vi "测试类型1自动测试一组.vi"() -> ()   [LabVIEW 2010]
uses:
  全局量/试验配置信息.vi
  全局量/自动测试结果.vi
panel:
  out "EVENT_KEY":string
  out "bRece":bool
  out "bSend":bool
  out "第几个":i32
  in  "测试值":dbl
  out "bStop":bool
  out "数据组数":i32
  out "第几组":i32
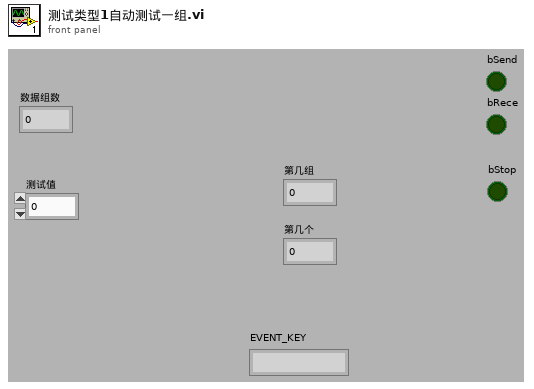
[diagram p1: front panel]
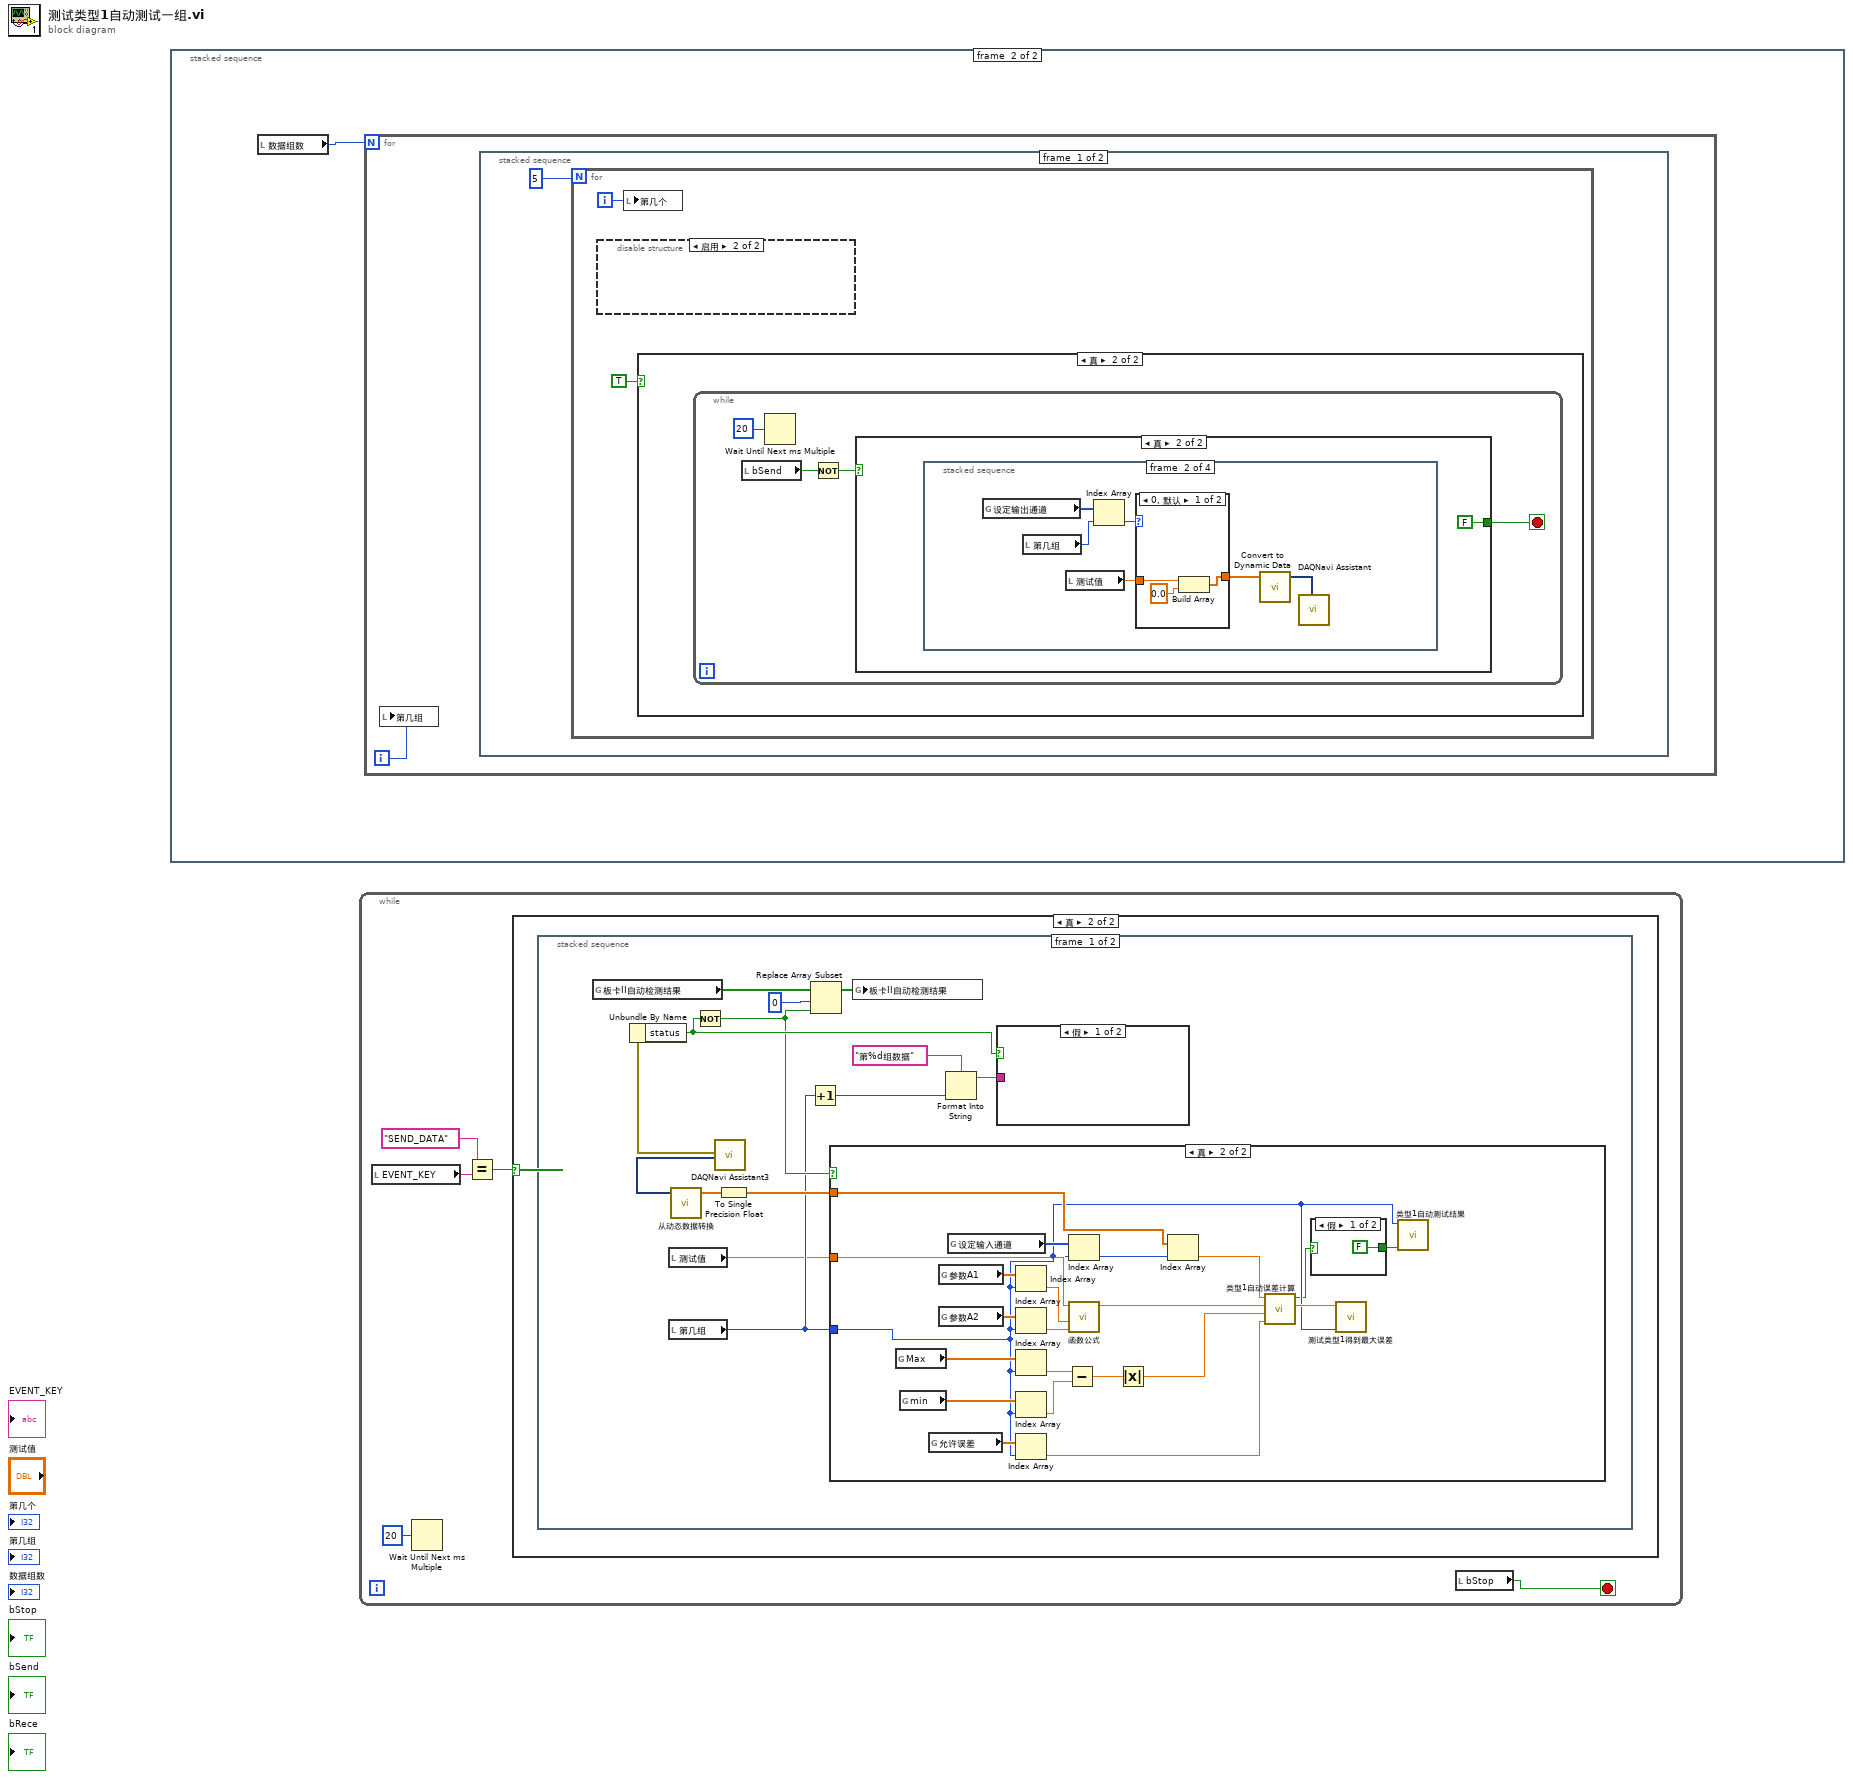
[diagram p0: block diagram]
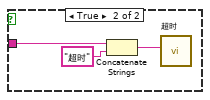
[diagram p3: hidden frame]
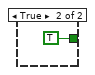
[diagram p5: hidden frame]
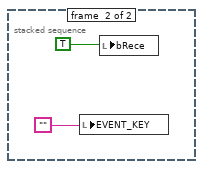
[diagram p6: hidden frame]
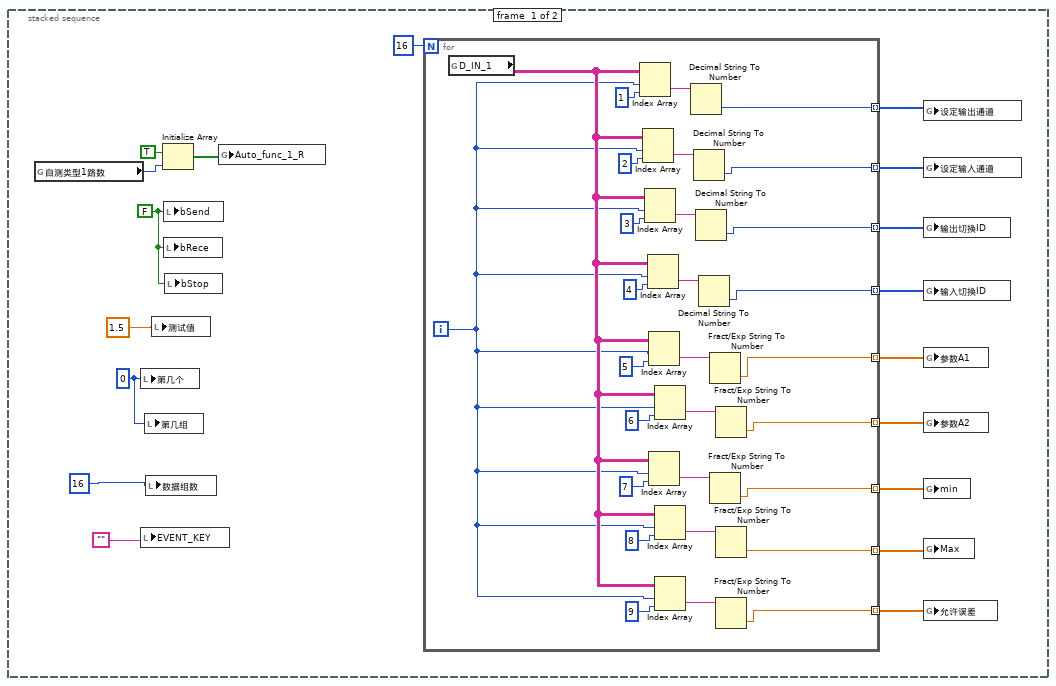
[diagram p7: hidden frame]
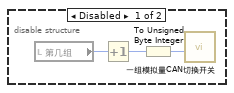
[diagram p8: hidden frame]
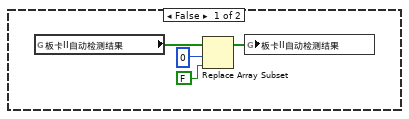
[diagram p9: hidden frame]
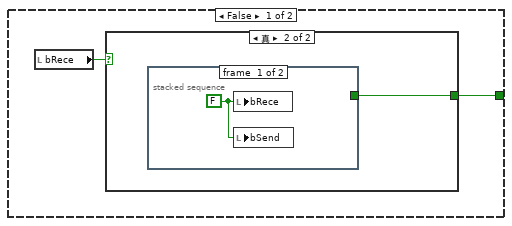
[diagram p10: hidden frame]
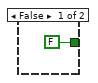
[diagram p11: hidden frame]
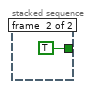
[diagram p12: hidden frame]
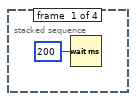
[diagram p13: hidden frame]
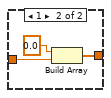
[diagram p14: hidden frame]
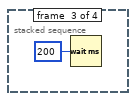
[diagram p15: hidden frame]
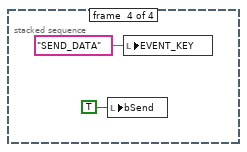
[diagram p16: hidden frame]
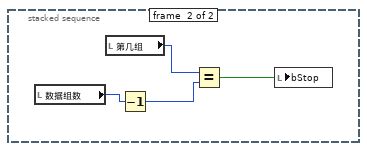
[diagram p17: hidden frame]
diagram:
  n1 = stacked-sequence {
    frame #0 {
      w12 = FALSE
      w17 = 0 ("同步A")
      n2 = global read "试验配置信息.vi" "自测类型1路数"() -> (w14:i32)
      n3 = local write "第几个"(w17) -> ()
      n4 = local write "EVENT_KEY"("") -> ()
      n5 = local write "第几组"(w17) -> ()
      n6 = local write "数据组数"(16) -> ()
      n7 = local write "测试值"(1.5 ("数值")) -> ()
      n8 = Initialize Array(TRUE ("元素"), w14) -> (w13:bool[])
      n9 = local write "bSend"(w12) -> ()
      n10 = local write "bRece"(w12) -> ()
      n11 = local write "bStop"(w12) -> ()
      n12 = global write "自动测试结果.vi" "Auto_func_1_R"(w13) -> ()
      n13 = for {
        N: 16 ("维数大小") -> [_]
        tunnel: [w27] -> w2 mode=indexing
        tunnel: [w26] -> w3 mode=indexing
        tunnel: [w25] -> w4 mode=indexing
        tunnel: [w24] -> w5 mode=indexing
        tunnel: [w23] -> w6 mode=indexing
        tunnel: [w22] -> w7 mode=indexing
        tunnel: [w21] -> w8 mode=indexing
        tunnel: [w20] -> w9 mode=indexing
        tunnel: [w19] -> w10 mode=indexing
        i -> [w28]
        n14 = global read "试验配置信息.vi" "D_IN_1"() -> (w29:string[][])
        n15 = Index Array(array=w29, index (row)=w28, index (col)=1 ("禁用的索引 (列)")) -> (element=w47:string)
        n16 = Index Array(array=w29, index (row)=w28, index (col)=2 ("禁用的索引 (列)")) -> (element=w44:string)
        n17 = Index Array(array=w29, index (row)=w28, index (col)=3 ("禁用的索引 (列)")) -> (element=w40:string)
        n18 = Index Array(array=w29, index (row)=w28, index (col)=4 ("禁用的索引 (列)")) -> (element=w43:string)
        n19 = Index Array(array=w29, index (row)=w28, index (col)=5 ("禁用的索引 (列)")) -> (element=w38:string)
        n20 = Index Array(array=w29, index (row)=w28, index (col)=7 ("禁用的索引 (列)")) -> (element=w33:string)
        n21 = Index Array(array=w29, index (row)=w28, index (col)=6 ("禁用的索引 (列)")) -> (element=w37:string)
        n22 = Index Array(array=w29, index (row)=w28, index (col)=8 ("禁用的索引 (列)")) -> (element=w34:string)
        n23 = Index Array(array=w29, index (row)=w28, index (col)=9 ("禁用的索引 (列)")) -> (element=w31:string)
        n24 = Decimal String To Number(string=w47) -> (number=w27:i32)  [unwired: 2 in, 1 out]
        n25 = Decimal String To Number(string=w44) -> (number=w26:i32)  [unwired: 2 in, 1 out]
        n26 = Decimal String To Number(string=w40) -> (number=w25:i32)  [unwired: 2 in, 1 out]
        n27 = Decimal String To Number(string=w43) -> (number=w24:i32)  [unwired: 2 in, 1 out]
        n28 = Fract/Exp String To Number(string=w38) -> (number=w23:dbl)  [unwired: 3 in, 1 out]
        n29 = Fract/Exp String To Number(string=w33) -> (number=w21:dbl)  [unwired: 3 in, 1 out]
        n30 = Fract/Exp String To Number(string=w37) -> (number=w22:dbl)  [unwired: 3 in, 1 out]
        n31 = Fract/Exp String To Number(string=w34) -> (number=w20:dbl)  [unwired: 3 in, 1 out]
        n32 = Fract/Exp String To Number(string=w31) -> (number=w19:dbl)  [unwired: 3 in, 1 out]
      }
      n33 = global write "试验配置信息.vi" "设定输出通道"(w2) -> ()
      n34 = global write "试验配置信息.vi" "设定输入通道"(w3) -> ()
      n35 = global write "试验配置信息.vi" "输出切换ID"(w4) -> ()
      n36 = global write "试验配置信息.vi" "输入切换ID"(w5) -> ()
      n37 = global write "试验配置信息.vi" "参数A1"(w6) -> ()
      n38 = global write "试验配置信息.vi" "参数A2"(w7) -> ()
      n39 = global write "试验配置信息.vi" "min"(w8) -> ()
      n40 = global write "试验配置信息.vi" "Max"(w9) -> ()
      n41 = global write "试验配置信息.vi" "允许误差"(w10) -> ()
    }
    frame #1 {
      n42 = local read "数据组数"() -> (w48:i32)
      n43 = for {
        N: w48 -> [_]
        i -> [w49]
        n44 = local write "第几组"(w49) -> ()
        n45 = stacked-sequence {
          frame #0 {
            n46 = for {
              N: 5 -> [_]
              i -> [w52]
              n47 = disable-structure shown="启用" {
                frame Disabled {
                  n48 = local read "第几组"() -> (w53:i32)
                  n49 = Increment(x=w53) -> (x+1=w54:i32)
                  n50 = To Unsigned Byte Integer(number=w54) -> (unsigned 8bit integer=w55:u8)
                  n51 = call "一组模拟量CAN切换开关.vi"("第几组数据"=w55) -> ()  [unwired: 10 in, 1 out]
                }
                frame Enabled {
                }
              }
              n52 = local write "第几个"(w52) -> ()
              n53 = case shown="真" TRUE {
                frame False {
                  n54 = global read "试验配置信息.vi" "板卡II自动检测结果"() -> (w59:bool[])
                  n55 = Replace Array Subset(array=w59, new element=FALSE, index=0 ("索引")) -> (w58:bool[])
                  n56 = global write "试验配置信息.vi" "板卡II自动检测结果"(w58) -> ()
                }
                frame True {
                  n57 = while {
                    stop <- w61 stop-if-true
                    n58 = local read "bSend"() -> (w63:bool)
                    n59 = Wait Until Next ms Multiple(millisecond multiple=u32 20 ("毫秒倍数")) -> ()  [unwired: 1 out]
                    n60 = Not(x=w63) -> (.not. x?=w62:bool)
                    n61 = case shown="真" w62 {
                      tunnel: [w64 FALSE] -> w61
                      frame False {
                        n62 = local read "bRece"() -> (w65:bool)
                        n63 = case shown="真" w65 {
                          tunnel: [FALSE w67] -> w64
                          frame False {
                          }
                          frame True {
                            n64 = stacked-sequence {
                              tunnel: [_ TRUE] -> w67
                              frame #0 {
                                w68 = FALSE
                                n65 = local write "bRece"(w68) -> ()
                                n66 = local write "bSend"(w68) -> ()
                              }
                              frame #1 {
                              }
                            }
                          }
                        }
                      }
                      frame True {
                        n67 = stacked-sequence {
                          frame #0 {
                            n68 = Wait (ms)(milliseconds to wait=u32 200 ("等待时间（毫秒）")) -> ()  [unwired: 1 out]
                          }
                          frame #1 {
                            n69 = global read "试验配置信息.vi" "设定输出通道"() -> (w73:i32[])
                            n70 = local read "第几组"() -> (w76:i32)
                            n71 = local read "测试值"() -> (w77:dbl)
                            n72 = Index Array(array=w73, index=w76) -> (element=w74:i32)
                            n73 = case shown="0, 默认" w74 {
                              tunnel: [w80 w83] -> w75
                              tunnel: w77 -> [w78 w81]
                              frame 0, Default {
                                n74 = Build Array(w78, 0.0) -> (w80:dbl[])
                              }
                              frame 1 {
                                n75 = Build Array(0.0, w81) -> (w83:dbl[])
                              }
                            }
                            n76 = call "Convert to Dynamic Data"("Array"=w75) -> ("Dynamic Data Type"=w72:dynamicdata)  [unwired: 3 out]
                            n77 = call "DAQNavi Assistant"("data in(DDT)"=w72) -> ()  [unwired: 2 in, 17 out]
                          }
                          frame #2 {
                            n78 = Wait (ms)(milliseconds to wait=u32 200 ("等待时间（毫秒）")) -> ()  [unwired: 1 out]
                          }
                          frame #3 {
                            n79 = local write "bSend"(TRUE) -> ()
                            n80 = local write "EVENT_KEY"("SEND_DATA" ("EVENT_KEY")) -> ()
                          }
                        }
                      }
                    }
                  }
                }
              }
            }
          }
          frame #1 {
            n81 = local read "数据组数"() -> (w88:i32)
            n82 = local read "第几组"() -> (w90:i32)
            n83 = Decrement(x=w88) -> (x-1=w87:i32)
            n84 = Equal?(x=w90, y=w87) -> (x = y?=w89:bool)
            n85 = local write "bStop"(w89) -> ()
          }
        }
      }
    }
  }
  n86 = while {
    stop <- w91 stop-if-true
    n87 = local read "EVENT_KEY"() -> (w94:string)
    n88 = Wait Until Next ms Multiple(millisecond multiple=u32 20 ("毫秒倍数")) -> ()  [unwired: 1 out]
    n89 = Equal?(x="SEND_DATA" ("EVENT_KEY"), y=w94) -> (x = y?=w93:bool)
    n90 = case shown="真" w93 {
      frame False {
      }
      frame True {
        n91 = stacked-sequence {
          frame #0 {
            n92 = global read "试验配置信息.vi" "板卡II自动检测结果"() -> (w103:bool[])
            n93 = local read "测试值"() -> (w96:dbl)
            n94 = local read "第几组"() -> (w97:i32)
            n95 = call "DAQNavi Assistant3"() -> ("error out"=w105:errorcluster, "data out(DDT)"=w106:dynamicdata)  [unwired: 2 in, 16 out]
            n96 = Unbundle By Name(w105) -> ("status"=w109:bool)
            n97 = call "从动态数据转换"("Dynamic Data Type"=w106) -> ("Array"=w107:dbl[])  [unwired: 3 in]
            n98 = Not(x=w109) -> (.not. x?=w104:bool)
            n99 = To Single Precision Float(number=w107) -> (single precision float=w108:sgl[])
            n100 = Increment(x=w97) -> (x+1=w100:i32)
            n101 = Replace Array Subset(array=w103, new element=w104, index=0 ("索引")) -> (w102:bool[])
            n102 = case shown="真" w104 {
              tunnel: w96 -> [_ w134]
              tunnel: w108 -> [_ w131]
              tunnel: w97 -> [_ w116]
              frame False {
              }
              frame True {
                n103 = global read "试验配置信息.vi" "Max"() -> (w127:dbl[])
                n104 = global read "试验配置信息.vi" "min"() -> (w128:dbl[])
                n105 = global read "试验配置信息.vi" "允许误差"() -> (w126:dbl[])
                n106 = global read "试验配置信息.vi" "参数A1"() -> (w130:dbl[])
                n107 = global read "试验配置信息.vi" "参数A2"() -> (w129:dbl[])
                n108 = global read "试验配置信息.vi" "设定输入通道"() -> (w133:i32[])
                n109 = Index Array(array=w130, index=w116) -> (element=w118:dbl)
                n110 = Index Array(array=w129, index=w116) -> (element=w122:dbl)
                n111 = Index Array(array=w127, index=w116) -> (element=w124:dbl)
                n112 = Index Array(array=w128, index=w116) -> (element=w123:dbl)
                n113 = Index Array(array=w126, index=w116) -> (element=w121:dbl)
                n114 = Subtract(x=w124, y=w123) -> (x-y=w125:dbl)
                n115 = Index Array(array=w133, index=w116) -> (element=w132:i32)
                n116 = call "函数公式.vi"("参数 b"=w122, "参数 a"=w118, "设定值 1"=w134) -> ("y"=w114:dbl)  [unwired: 5 in, 1 out]
                n117 = Absolute Value(x=w125) -> (abs(x)=w117:dbl)
                n118 = Index Array(array=w131, index=w132) -> (element=w115:sgl)
                n119 = call "类型1自动误差计算.vi"("允许误差"=w121, "模拟量量程范围"=w117, "设定值_1"=w114, "反馈值_1"=w115) -> ("误差_1"=w119:dbl, "合格_1?"=w113:bool)  [unwired: 5 in, 1 out]
                n120 = case shown="假" w113 {
                  tunnel: [FALSE TRUE] -> w120
                  frame False {
                  }
                  frame True {
                  }
                }
                n121 = call "测试类型1得到最大误差.vi"("第几组"=w116, "新误差值"=w119) -> ()  [unwired: 10 in]
                n122 = call "类型1自动测试结果.vi"("合格?"=w120, "第几组"=w116) -> ()  [unwired: 10 in]
              }
            }
            n123 = global write "试验配置信息.vi" "板卡II自动检测结果"(w102) -> ()
            n124 = Format Into String(format string="第%d组数据" ("格式字符串"), w100) -> (resulting string=w99:string)  [unwired: 2 in, 1 out]
            n125 = case shown="假" w109 {
              tunnel: w99 -> [_ w112]
              frame False {
              }
              frame True {
                n126 = Concatenate Strings(w112, "超时" ("格式字符串")) -> (w110:string)
                n127 = call "超时"("Message"=w110) -> ()  [unwired: 9 in, 2 out]
              }
            }
          }
          frame #1 {
            n128 = local write "EVENT_KEY"("") -> ()
            n129 = local write "bRece"(TRUE) -> ()
          }
        }
      }
    }
    n130 = local read "bStop"() -> (w91:bool)
  }
